vi "FIFOMultiChannelToHost.vi"(8 "Reset":bool, 9 "FIFO control":T1, 11 "Multi Channel Data":T2={"Multi Channel Data"=[0, 0, 0, 0], "Data Valid"=FALSE, "Pixel Overwritten by Tag"=FALSE}) -> (0 "FIFO Multi Channels Pixels Lost":u32, 2 "assert pixel overwritten interrupt":bool, 3 "assert FIFO overflow interrupt":bool)   [LabVIEW 2014]
uses:
  <vilib>/rvi/DataTransferAndStorage/Container/XNode/niFpgaContainer.xnode
  <vilib>/rvi/interface/RandomDataEmulation/nirviRandomDataFpgaReadWriteTemplate.vi
panel:
  # "Copyright 2014 Vidrio Technologies\nScanImage 5 software is licensed under the Apache License, Version 2.0 (the \"License\"); you may not use any files contained\nwithin the ScanImage 5 release except in compliance with the License. You may obtain a copy of the License at\n http://www.apache.org/licenses/LICENSE-2.0\nUnless required by applicable law or agreed to in writing, software distributed under the License is distributed on an\n\"AS IS\" BASIS, WITHOUT WARRANTIES OR CONDITIONS OF ANY KIND, either express or implied. See the License for the\n specific language governing permissions and limitations under the License."
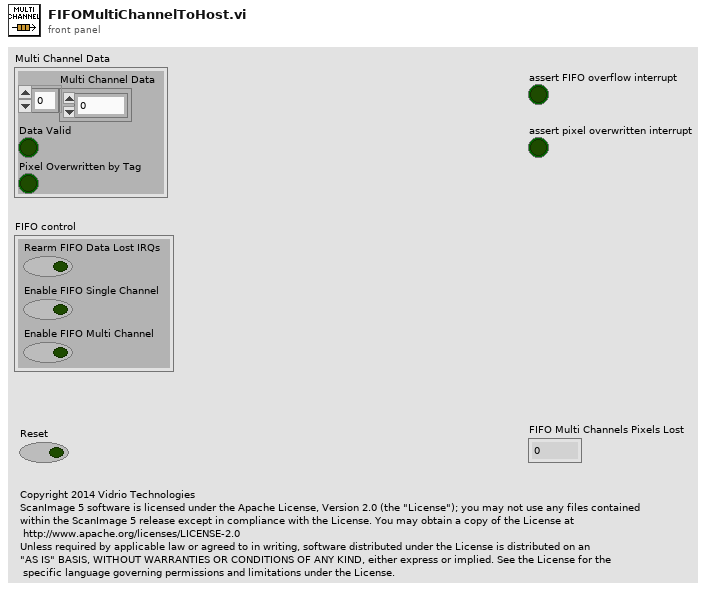
[diagram p1: front panel]
types:
  T1 = cluster{"Rearm FIFO Data Lost IRQs":bool, "Enable FIFO Single Channel":bool, "Enable FIFO Multi Channel":bool}
  T2 = cluster{"Multi Channel Data":i16[], "Data Valid":bool, "Pixel Overwritten by Tag":bool}
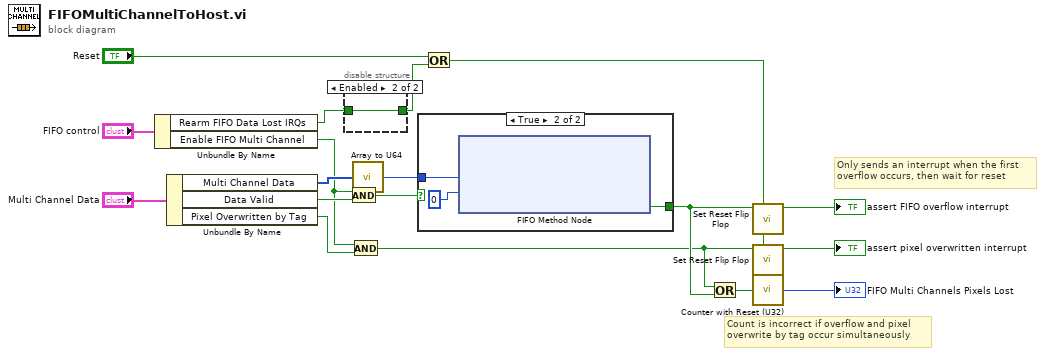
[diagram p0: block diagram]
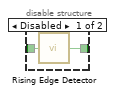
[diagram p2: hidden frame]
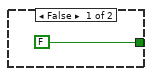
[diagram p3: hidden frame]
diagram:
  # "Count is incorrect if overflow and pixel\noverwrite by tag occur simultaneously"
  # "Only sends an interrupt when the first\noverflow occurs, then wait for reset"
  n1 = Unbundle By Name("FIFO control") -> ("Rearm FIFO Data Lost IRQs"=w2:bool, "Enable FIFO Multi Channel"=w8:bool)
  n2 = Unbundle By Name("Multi Channel Data") -> ("Multi Channel Data"=w13:i16[], "Data Valid"=w10:bool, "Pixel Overwritten by Tag"=w7:bool)
  n3 = disable-structure shown="Enabled" {
    disable-tunnel: w2 -> [w20 w21]
    disable-tunnel: [w19 w21] -> w1
    frame Disabled {
      n4 = call "Rising Edge Detector.vi"("signal"=w20) -> ("edge detected"=w19:bool)  [unwired: 14 in]
    }
    frame Enabled {
    }
  }
  n5 = And(x=w8, y=w10) -> (x .and. y?=w17:bool)
  n6 = And(x=w8, y=w7) -> (x .and. y?=w4:bool)
  n7 = call "Array to U64.vi"("Input Array I16"=w13) -> ("Output U64"=w16:u64)  [unwired: 14 in]
  n8 = case shown="True" w17 {
    tunnel: [FALSE ("Timed Out?") w25] -> w5
    tunnel: w16 -> [_ w23]
    frame False {
    }
    frame True {
      n9 = xnode ("FIFO Method Node")("Element"=w23, "Timeout"=0) -> ("Timed Out?"=w25:bool)  [unwired: 1 in, 1 out]
    }
  }
  n10 = Or(x="Reset", y=w1) -> (x .or. y?=w9:bool)
  n11 = Or(x=w4, y=w5) -> (x .or. y?=w6:bool)
  n12 = call "Set Reset Flip Flop.vi"("Reset"=w9, "Set"=w5) -> ("Out"=→"assert FIFO overflow interrupt":bool)  [unwired: 9 in]
  n13 = call "Set Reset Flip Flop.vi"("Reset"=w9, "Set"=w4) -> ("Out"=→"assert pixel overwritten interrupt":bool)  [unwired: 9 in]
  n14 = call "Counter with Reset (U32).vi"("Reset?"=w9, "Increment"=w6) -> ("Counter"=→"FIFO Multi Channels Pixels Lost":u32)  [unwired: 13 in]
